vi "Acciones_Mecanicas.vi"() -> ()   [LabVIEW 2016]
panel:
  out "Boolean 2":bool
  in  "Boolean":bool
  in  "Stop Button":bool
  # "Mechanical Action"
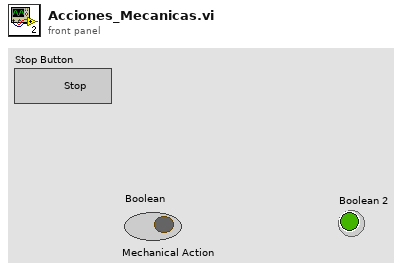
[diagram p1: front panel]
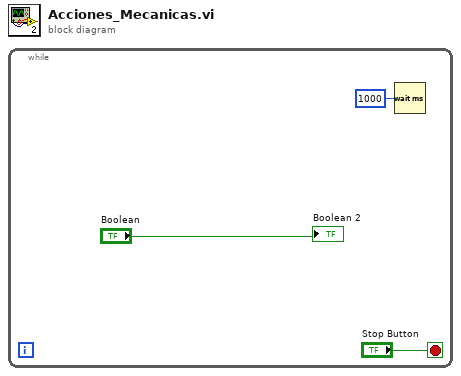
[diagram p0: block diagram]
diagram:
  n1 = while {
    stop <- "Stop Button" stop-if-true
    n2 = Wait (ms)(milliseconds to wait=u32 1000) -> ()  [unwired: 1 out]
    "Boolean 2" <- "Boolean"
  }
